vi "Conditional Invert.vi"(2 "x":dbl, 3 "invert":bool) -> (0 "invert ? x : -x":dbl)   [LabVIEW 2012]
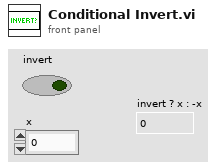
[diagram p1: front panel]
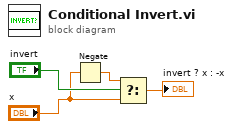
[diagram p0: block diagram]
diagram:
  n1 = Negate(x="x") -> (-x=w2:dbl)
  n2 = Select(t=w2, s="invert", f="x") -> (s? t:f=→"invert ? x : -x":dbl)
